vi "Counter - Read Encoder Velocity3 (Continuous Clock).vi"() -> ()   [LabVIEW 2015]
doc: "This example demonstrates how to use a counter input along with an external clock to continually sample the angular velocity measured from an encoder.\n\nFor instructions on how to connect your signals to the DAQ device, refer to your device documentation."
uses:
  <resource>/objmgr/daqmx.rc
  <vilib>/DAQmx/configure/timing.llb/DAQmx Timing (Sample Clock).vi
  <vilib>/Utility/error.llb/DialogType.ctl
  <vilib>/DAQmx/create/channels.llb/DAQmx Create Channel (AI-Voltage-Basic).vi
  <vilib>/DAQmx/create/channels.llb/DAQmx Create Channel (CI-Velocity-Linear).vi
  <vilib>/DAQmx/read.llb/DAQmx Read (Analog 1D Wfm NChan NSamp).vi
  <vilib>/DAQmx/read.llb/DAQmx Read (Counter 2D DBL NChan NSamp).vi
panel:
  in  "Channel 2":bool=TRUE
  in  "Channel 1":bool=TRUE
  out "appended path":path
  in  "Row 1 Header":string="Header Information Row 1"
  out "Boolean":bool
  out "Waveform Chart":dbl(graph)
  out "Numeric Indicator":dbl format="%#_4g"
  in  "Counter 0":tag="Mantis1_1Mod4/ctr0"
  in  "B Input Terminal":tag="/Mantis1_1Mod4/PFI7"
  in  "A Input Terminal":tag="/Mantis1_1Mod4/PFI0"
  in  "Stop":bool
  in  "Samples per Loop":i32=1
  in  "Sample Rate":dbl=100.0
  in  "Sample Clock Source":tag="OnboardClock"
  # "MPH"
  # "Channel Settings"
  # "Saving data"
  # "Timing Settings"
  # "Trigger Rising Edge?"
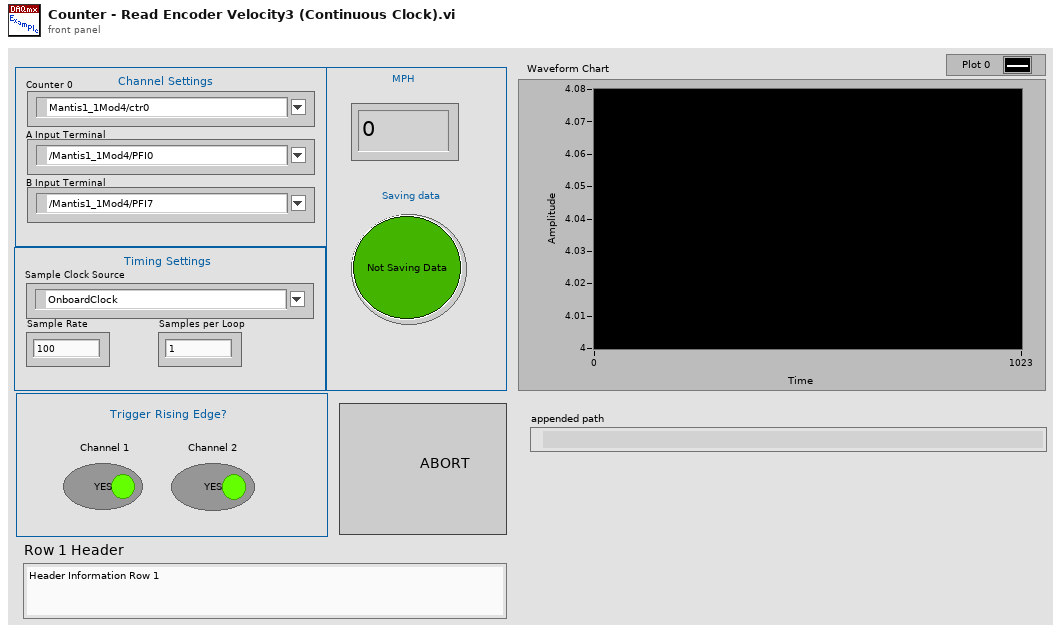
[diagram p1: front panel]
types:
  T1 = typedef "DialogType.ctl" = u16
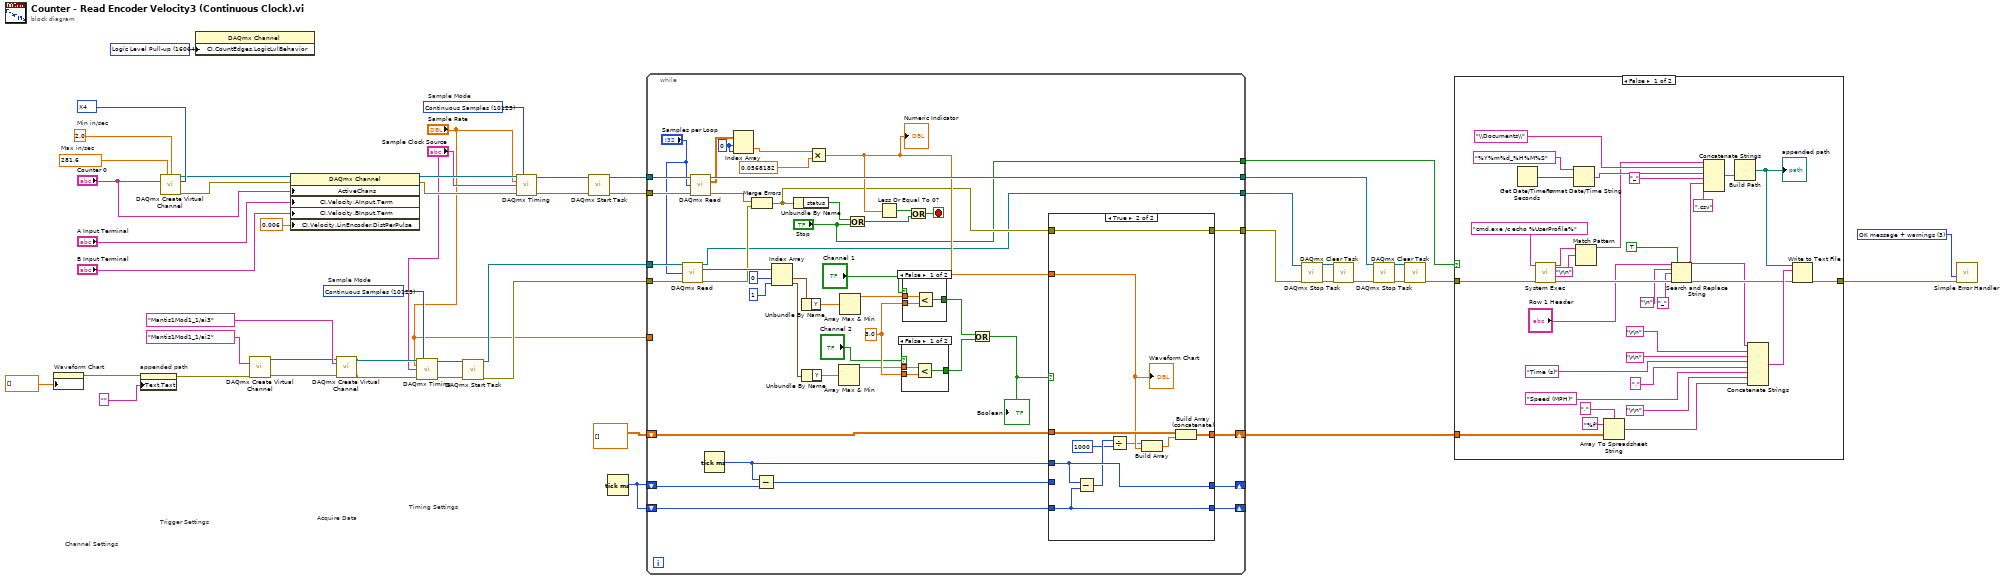
[diagram p0: block diagram]
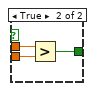
[diagram p3: hidden frame]
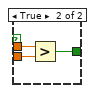
[diagram p4: hidden frame]
diagram:
  w1 = 16064 items=["Logic Level Pull-up"=16064, "None"=10230] ("CI.CountEdges.LogicLvlBehavior")
  w27 = 10123 items=["Finite Samples"=10178, "Continuous Samples"=10123, "Hardware Timed Single Point"=12522]  # Sample Mode
  w42 = 281.6  # Max in/sec
  w41 = 2.0  # Min in/sec
  w36 = 10092 items=["X1"=10090, "X2"=10091, "X4"=10092, "Two Pulse Counting"=10313] ("decoding type")
  w44 = T1 3 items=["no dialog", "OK message", "continue or stop message", "OK message + warnings", "continue/stop + warnings"] ("type of dialog (OK msg:1)")
  w49 = 10123 items=["Finite Samples"=10178, "Continuous Samples"=10123, "Hardware Timed Single Point"=12522]  # Sample Mode
  # "Acquire Data"
  # "Trigger Settings"
  # "Timing Settings"
  # "Channel Settings"
  n1 = property on="Waveform Chart" class="WFChart (strict)"("History Data"=dbl[] []) -> (error out=w12:errorcluster)  [unwired: 2 in, 1 out]
  n2 = property on="appended path" class="Path"(error in=w12, "Text.Text"="" ("Path Text.Text")) -> (error out=w11:errorcluster)  [unwired: 1 in, 1 out]
  n3 = call-poly <vilib>:"DAQmx Create Virtual Channel.vi"("maximum value"=w42, "minimum value"=w41, "counter"="Counter 0", "decoding type"=w36) -> ("task out"=w2:refnum<k21>, "error out"=w43:errorcluster)  [unwired: 10 in]
  n4 = property class="DAQmx Channel"("CI.CountEdges.LogicLvlBehavior"=w1) -> ()  [unwired: 2 in, 2 out]
  n5 = call-poly <vilib>:"DAQmx Create Virtual Channel.vi"("physical channels"=tag "Mantis1Mod1_1/ai2", "error in"=w11) -> ("task out"=w33:refnum<k21>, "error out"=w32:errorcluster)  [unwired: 12 in]
  n6 = property class="DAQmx Channel"(reference=w2, error in=w43, "ActiveChans"="Counter 0", "CI.Velocity.AInput.Term"="A Input Terminal", "CI.Velocity.BInput.Term"="B Input Terminal", "CI.Velocity.LinEncoder.DistPerPulse"=0.006) -> (reference out=w30:refnum<k21>, error out=w31:errorcluster)
  n7 = call-poly <vilib>:"DAQmx Create Virtual Channel.vi"("task in"=w33, "physical channels"=tag "Mantis1Mod1_1/ai3", "error in"=w32) -> ("task out"=w26:refnum<k21>, "error out"=w25:errorcluster)  [unwired: 11 in]
  n8 = call-poly <vilib>:"DAQmx Timing.vi"("task/channels in"=w26, "sample mode"=w27, "rate"="Sample Rate", "source"="Sample Clock Source", "error in"=w25) -> ("task out"=w23:refnum<k21>, "error out"=w22:errorcluster)  [unwired: 9 in]
  n9 = call <vilib>:"DAQmx Start Task.vi"("task/channels in"=w23, "error in"=w22) -> ("task out"=w20:refnum<k21>, "error out"=w19:errorcluster)  [unwired: 12 in]
  n10 = call-poly <vilib>:"DAQmx Timing.vi"("task/channels in"=w30, "sample mode"=w49, "rate"="Sample Rate", "source"="Sample Clock Source", "error in"=w31) -> ("task out"=w28:refnum<k21>, "error out"=w29:errorcluster)  [unwired: 9 in]
  n11 = call <vilib>:"DAQmx Start Task.vi"("task/channels in"=w28, "error in"=w29) -> ("task out"=w48:refnum<k21>, "error out"=w47:errorcluster)  [unwired: 12 in]
  n12 = Tick Count (ms)() -> (millisecond timer value=w13:u32)
  n13 = while {
    tunnel: w48 -> [w93]
    tunnel: w47 -> [w92]
    tunnel: [w91] -> w6
    tunnel: w20 -> [w75]
    tunnel: w19 -> [w74]
    tunnel: "Sample Rate" -> [_]
    shift-right: [w65] -> _
    shift-left: w13 -> [w64]
    shift-right: [w57] -> _
    shift-left: w13 -> [w58]
    shift-right: [w55] -> w16
    shift-left: dbl[][] [] -> [w56]
    tunnel: [w54] -> w4
    tunnel: [w51] -> w5
    tunnel: ["Stop"] -> w3
    stop <- w71 stop-if-true
    w84 = 3.0 ("y")
    w69 = 0 ("disabled index (col)")
    n14 = call-poly <vilib>:"DAQmx Read.vi"("task/channels in"=w75, "number of samples per channel"="Samples per Loop", "error in"=w74) -> ("task out"=w51:refnum<k21>, "data"=w87:waveform(dbl)[], "error out"=w62:errorcluster)  [unwired: 10 in]
    n15 = call-poly <vilib>:"DAQmx Read.vi"("task/channels in"=w93, "number of samples per channel"="Samples per Loop", "error in"=w92) -> ("task out"=w91:refnum<k21>, "data"=w89:dbl[][], "error out"=w61:errorcluster)  [unwired: 10 in]
    n16 = Tick Count (ms)() -> (millisecond timer value=w63:u32)
    n17 = Index Array(array=w89, index (row)=w69, index (col)=w69) -> (element=w68:dbl)
    n18 = Merge Errors(w61, w62) -> (w60:errorcluster)
    n19 = Subtract(x=w63, y=w64) -> (x-y=w59:u32)
    n20 = Index Array(array=w87, index #1=0 ("index"), index #2=1 ("index")) -> (element #1=w77:waveform(dbl), element #2=w80:waveform(dbl))
    n21 = Unbundle By Name(w60) -> ("status"=w90:bool)
    n22 = Unbundle By Name(w77) -> ("Y"=w78:dbl[])
    n23 = Unbundle By Name(w80) -> ("Y"=w81:dbl[])
    n24 = Multiply(x=w68, y=0.0568182) -> (x*y=w70:dbl)
    "Numeric Indicator" <- w70
    n25 = Array Max & Min(array=w81) -> (max value=w83:dbl)  [unwired: 3 out]
    n26 = Array Max & Min(array=w78) -> (max value=w82:dbl)  [unwired: 3 out]
    n27 = Or(x=w90, y="Stop") -> (x .or. y?=w73:bool)
    n28 = Less Or Equal To 0?(x=w70) -> (x <= 0?=w72:bool)
    n29 = case shown="False" "Channel 2" {
      tunnel: [w95 w99] -> w86
      tunnel: w84 -> [w96 w98]
      tunnel: w83 -> [w94 w97]
      frame False {
        n30 = Less?(x=w94, y=w96) -> (x < y?=w95:bool)
      }
      frame True {
        n31 = Greater?(x=w97, y=w98) -> (0:w99:bool)
      }
    }
    n32 = case shown="False" "Channel 1" {
      tunnel: [w102 w105] -> w85
      tunnel: w84 -> [w100 w104]
      tunnel: w82 -> [w101 w103]
      frame False {
        n33 = Less?(x=w101, y=w100) -> (x < y?=w102:bool)
      }
      frame True {
        n34 = Greater?(x=w103, y=w104) -> (0:w105:bool)
      }
    }
    n35 = Or(x=w72, y=w73) -> (x .or. y?=w71:bool)
    n36 = Or(x=w85, y=w86) -> (x .or. y?=w67:bool)
    "Boolean" <- w67
    n37 = case shown="True" w67 {
      tunnel: w70 -> [_ w115]
      tunnel: w63 -> [w106 w113]
      tunnel: [w106 w113] -> w65
      tunnel: w60 -> [w107 w114]
      tunnel: w59 -> [_ _]
      tunnel: w58 -> [_ w112]
      tunnel: [w106 w112] -> w57
      tunnel: [w108 w117] -> w55
      tunnel: w56 -> [w108 w118]
      tunnel: [w107 w114] -> w54
      frame False {
      }
      frame True {
        n38 = Subtract(x=w113, y=w112) -> (x-y=w110:u32)
        n39 = Divide(x=w110, y=u32 1000) -> (x/y=w111:dbl)
        n40 = Build Array(w111, w115) -> (w116:dbl[])
        n41 = Build Array (concatenate)(w118, w116) -> (w117:dbl[][])
        "Waveform Chart" <- w115
      }
    }
  }
  n42 = call <vilib>:"DAQmx Stop Task.vi"("task/channels in"=w5, "error in"=w4) -> ("task out"=w9:refnum<k21>, "error out"=w8:errorcluster)  [unwired: 12 in]
  n43 = call <vilib>:"DAQmx Clear Task.vi"("task in"=w9, "error in"=w8) -> ("error out"=w7:errorcluster)  [unwired: 13 in]
  n44 = call <vilib>:"DAQmx Stop Task.vi"("task/channels in"=w6, "error in"=w7) -> ("task out"=w45:refnum<k21>, "error out"=w46:errorcluster)  [unwired: 12 in]
  n45 = call <vilib>:"DAQmx Clear Task.vi"("task in"=w45, "error in"=w46) -> ("error out"=w14:errorcluster)  [unwired: 13 in]
  n46 = case shown="False" w3 {
    tunnel: w16 -> [w145 _]
    tunnel: [w141 w151] -> w15
    tunnel: w14 -> [w131 w151]
    frame False {
      n47 = Get Date/Time In Seconds() -> (seconds since 1Jan1904=w139:timestamp)
      n48 = call <vilib>:"System Exec.vi"("error in (no error)"=w131, "command line"="cmd.exe /c echo %UserProfile%") -> ("error out"=w125:errorcluster, "standard output"=w130:string)  [unwired: 6 in, 2 out]
      n49 = Format Date/Time String(time format string (%c)="%Y%m%d_%H%M%S", seconds (now)=w139) -> (date/time string=w137:string)  [unwired: 1 out]
      n50 = Match Pattern(string=w130, regular expression="\r\n") -> (before substring=w129:string)  [unwired: 1 in, 3 out]
      n51 = Array To Spreadsheet String(delimiter (Tab)=",", array=w145, 3:"%f" ("format string")) -> (spreadsheet string=w142:string)
      n52 = Search and Replace String(replace all?=TRUE ("replace all? (F)"), input string="Row 1 Header", search string="\n", replace string="_" ("replace string (\"\")"), error in=w125) -> (result string=w122:string, error out=w124:errorcluster)  [unwired: 3 in, 2 out]
      n53 = Concatenate Strings(w129, "\\Documents\\" ("string"), w137, "_" ("string"), w122, ".csv" ("string")) -> (w136:string)
      n54 = Build Path(name or relative path=w136) -> (appended path=w135:path)  [unwired: 1 in]
      "appended path" <- w135
      n55 = Concatenate Strings(w122, "\r\n", "\r\n", "Time (s)", ",", "Speed (MPH)", "\r\n", w142) -> (w140:string)
      n56 = Write to Text File(file (use dialog)=w135, text=w140, error in=w124) -> (error out=w141:errorcluster)  [unwired: 1 in, 2 out]
    }
    frame True {
    }
  }
  n57 = call <vilib>:"Simple Error Handler.vi"("type of dialog (OK msg:1)"=w44, "error in (no error)"=w15) -> ()  [unwired: 3 in, 5 out]
